vi "Robot Global Data.vi"() -> ()   [LabVIEW 2011]
doc: "This global VI can contain as many global variables as you need. Place a control on the panel, give it a good name. To read or write to it from a VI, drag the icon to the diagram of that VI. You can also drag from the project. Click on the node to change which global you access. You shouldn't have multiple locations writing to a global or it will cause a race-condition."
uses:
  <vilib>/Rock Robotics/WPI/Camera/WPI_CameraImageSize.ctl
panel:
  out "Personality":string
  out "DEMO":bool
  in  "Tab Control":T1(tab)
  out "Kick Sonar":bool
  out "Op Button 12":bool
  out "Op Button 11":bool
  out "Op Button 1":bool
  out "Op Button 2":bool
  out "Op Button 3":bool
  out "Op Button 4":bool
  out "Op Button 5":bool
  out "Op Button 6":bool
  out "Op Button 7":bool
  out "Op Button 8":bool
  out "Op Button 9":bool
  out "Op Button 10":bool
  out "Dr Button 1":bool
  out "Dr Button 2":bool
  out "Dr Button 3":bool
  out "Dr Button 4":bool
  out "Dr Button 5":bool
  out "Dr Button 6":bool
  out "Dr Button 7":bool
  out "Dr Button 8":bool
  out "Dr Button 9":bool
  out "Dr Button 10":bool
  out "INTAKE Direction":bool
  out "Ball Count":dbl
  out "INTAKE":bool
  out "BB A/B":bool
  out "BB B":bool
  out "PRIME":bool
  out "Shooter RPM Offset":dbl
  out "Report Fire":bool
  out "Shooter RPM Tol":dbl
  out "Startup?":string
  out "Shooter RPM Control":dbl
  out "Shooter RPM Response":dbl
  out "Shooter Ready?":bool
  out "Shooter Stable?":bool
  out "Softstops Enabled":bool
  out "Turret Slow ?":bool
  out "Left_Limit":bool
  out "Right_Limit":bool
  out "Turret Yaw Joystick Command":dbl
  out "Turret Yaw Poition Command":dbl
  out "Turret Encoder":dbl
  out "Turret Yaw":dbl
  out "Turret Home":bool
  out "Turret Ready?":bool
  out "Turret Stable?":bool
  out "Turret Encoder Count":dbl
  out "Bridge is Down":bool
  out "Bridge is Up":bool
  out "Enable Fetch":bool
  out "Autonomous Drive":bool
  out "X Axis Drive Cmd":dbl
  out "Y Axis Drive Cmd":dbl
  out "Left Wheel Encoder":dbl
  out "Right Wheel Encoder":dbl
  out "Avg Wheel Encoder":dbl
  out "Pitch Gyro":dbl
  out "Compressor":bool
  out "Robot Gyro":dbl
  out "Robot Compass":dbl
  in  "TARGET AQUIRED":bool
  in  "FAILSAFE!":bool
  in  "Shooting Solution":bool
  out "Collector State Machine":bool
  out "Gear":u16(ring)=1 items=["HIGH", "LOW"]
  out "Auto Targeting ?":bool
  out "Auto Target":bool
  out "Target Bearing":dbl
  out "Turret SetPoint":dbl
  out "Valid Target ?":bool
  out "Frame Num":i32
  out "Fresh Target ?":bool
  out "Turret Position Command ?":bool
  out "Target Distance":dbl
  out "Target Angle":dbl
  out "Driver Turn to Target":dbl
  out "Target Info":T2(array[cluster])
  in  "LED toggle rate (ms)":u32=20
  in  "image size":T3=enum."320x240"
  in  "Enable Vision":bool
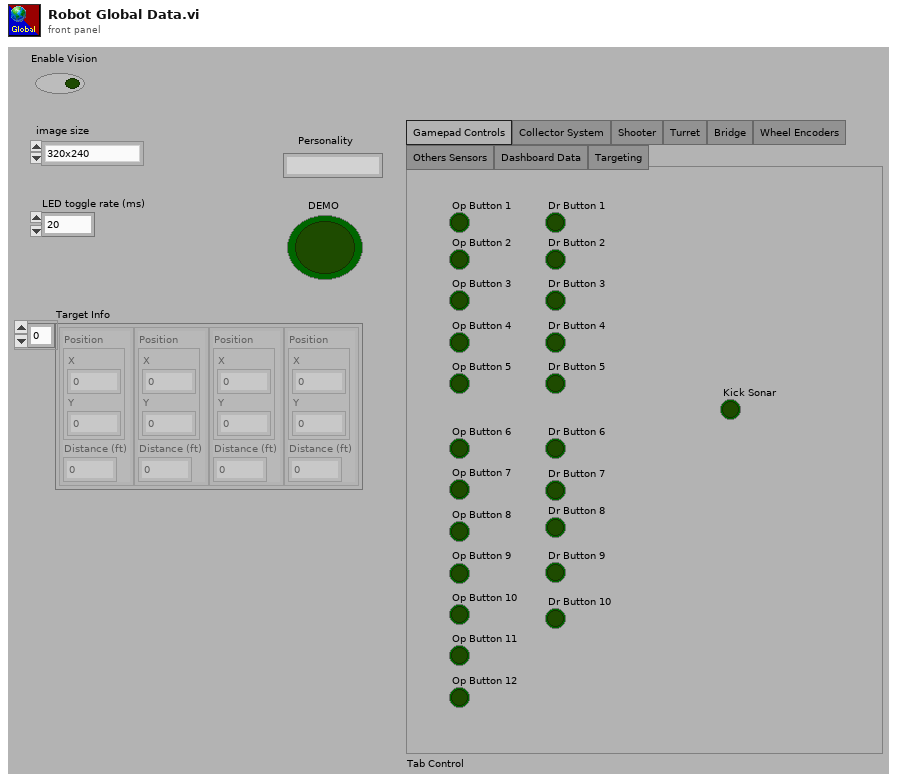
[diagram p1: front panel]
types:
  T1 = enum32{"Gamepad Controls", "Collector System", "Shooter", "Turret", "Bridge", "Wheel Encoders", "Others Sensors", "Dashboard Data", "Targeting"}
  T2 = cluster{"Position":cluster{"X":dbl, "Y":dbl}, "Distance (ft)":dbl}[]
  T3 = typedef "WPI_CameraImageSize.ctl" = enum16{"640x480", "320x240", "160x120"}
diagram:
